vi "Ctor.vi"(8 "error in (no error)":errorcluster, 11 "Ready Notifier":refnum<notifier>) -> (0 "error out":errorcluster, 3 "picoG out":refnum<class "picoG.lvclass">)   [LabVIEW 2020, in "PicoG-App.lvlib" / "picoG.lvclass"]
uses:
  picoG.lvclass
  Device/Device.lvclass
  picoG.lvclass/picoG.ctl
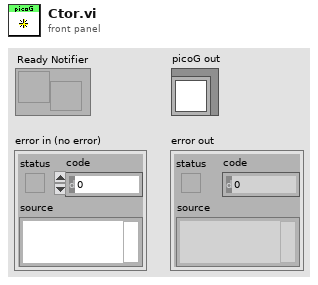
[diagram p1: front panel]
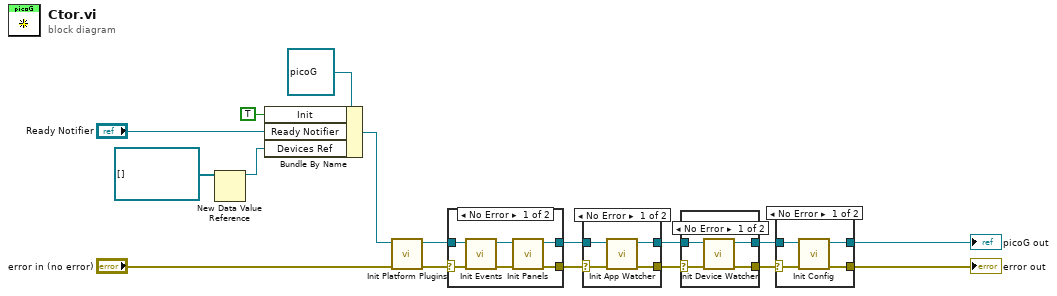
[diagram p0: block diagram]
diagram:
  n1 = New Data Value Reference(data value=refnum<class "Device.lvclass">[] []) -> (data value reference=w3:refnum<data-value>)  [unwired: 1 in, 1 out]
  n2 = Bundle By Name(cluster=refnum<class "picoG.lvclass"> refnum ("App in"), "Init"=TRUE, "Ready Notifier"="Ready Notifier", "Devices Ref"=w3) -> (w13:refnum<class "picoG.lvclass">)
  n3 = call "Init Platform Plugins.vi"("error in (no error)"="error in (no error)", "picoG in"=w13) -> ("error out"=w6:errorcluster, "picoG out"=w5:refnum<class "picoG.lvclass">)  [unwired: 8 in]
  n4 = case shown="No Error" w6 {
    selector: w6 -> [w23 w25]
    tunnel: w5 -> [w22 w24]
    tunnel: [w19 w24] -> w12
    tunnel: [w18 w25] -> w11
    frame No Error {
      n5 = call "Init Events.vi"("error in (no error)"=w23, "picoG in"=w22) -> ("error out"=w20:errorcluster, "picoG out"=w21:refnum<class "picoG.lvclass">)  [unwired: 8 in]
      n6 = call "Init Panels.vi"("error in (no error)"=w20, "picoG in"=w21) -> ("error out"=w18:errorcluster, "picoG out"=w19:refnum<class "picoG.lvclass">)  [unwired: 8 in]
    }
    frame Error {
    }
  }
  n7 = case shown="No Error" w11 {
    selector: w11 -> [w28 w30]
    tunnel: [w27 w30] -> w9
    tunnel: [w26 w31] -> w10
    tunnel: w12 -> [w29 w31]
    frame No Error {
      n8 = call "Init App Watcher.vi"("error in (no error)"=w28, "picoG in"=w29) -> ("error out"=w27:errorcluster, "picoG out"=w26:refnum<class "picoG.lvclass">)  [unwired: 8 in]
    }
    frame Error {
    }
  }
  n9 = case shown="No Error" w9 {
    selector: w9 -> [w35 w36]
    tunnel: [w32 w36] -> w8
    tunnel: [w33 w37] -> w7
    tunnel: w10 -> [w34 w37]
    frame No Error {
      n10 = call "Init Device Watcher.vi"("error in (no error)"=w35, "picoG in"=w34) -> ("error out"=w32:errorcluster, "picoG out"=w33:refnum<class "picoG.lvclass">)  [unwired: 8 in]
    }
    frame Error {
    }
  }
  n11 = case shown="No Error" w8 {
    selector: w8 -> [w39 w42]
    tunnel: [w41 w42] -> w1
    tunnel: [w40 w43] -> w2
    tunnel: w7 -> [w38 w43]
    frame No Error {
      n12 = call "Init Config.vi"("error in (no error)"=w39, "picoG in"=w38) -> ("error out"=w41:errorcluster, "picoG out"=w40:refnum<class "picoG.lvclass">)  [unwired: 8 in]
    }
    frame Error {
    }
  }
  "error out" <- w1
  "picoG out" <- w2
